vi "Write Action sequence.vi"(8 "error in (no error)":errorcluster, 10 "Action sequence":refnum<class "Action.lvclass">[](array[class]), 11 "Sequence in":refnum<class "Action-sequence.lvclass">) -> (0 "error out":errorcluster, 3 "Sequence out":refnum<class "Action-sequence.lvclass">)   [LabVIEW 2013, in "PowderDeposition.lvlib" / "Action-sequence.lvclass"]
uses:
  Action-sequence.lvclass
  Action/Action.lvclass
  Action-sequence.lvclass/Action-sequence.ctl
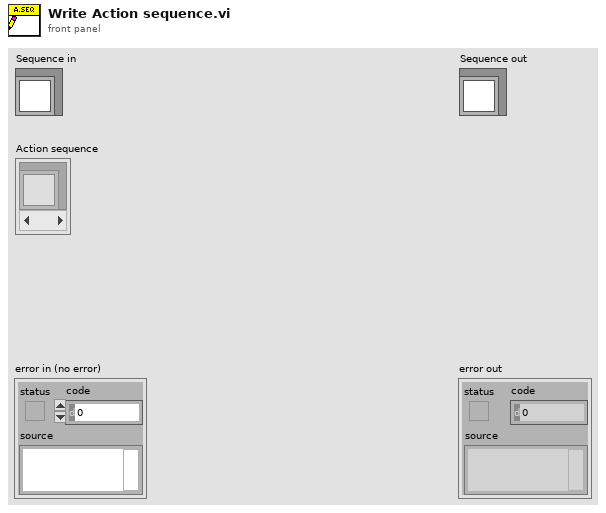
[diagram p1: front panel]
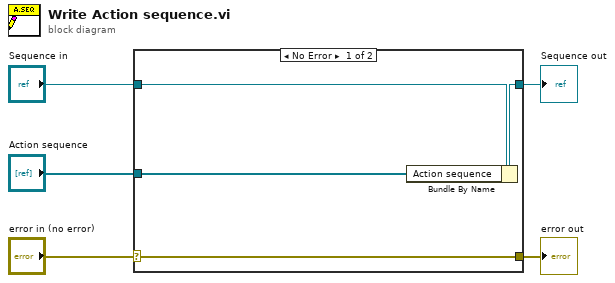
[diagram p0: block diagram]
diagram:
  n1 = case shown="No Error" "error in (no error)" {
    selector: "error in (no error)" -> [w9 w10]
    tunnel: [w9 w10] -> w4
    tunnel: [w7 w11] -> w2
    tunnel: "Sequence in" -> [w8 w11]
    tunnel: "Action sequence" -> [w6 _]
    frame No Error {
      n2 = Bundle By Name(cluster=w8, "Action sequence"=w6) -> (w7:refnum<class "Action-sequence.lvclass">)
    }
    frame Error {
    }
  }
  "error out" <- w4
  "Sequence out" <- w2
